vi "PH_Beckhoff.set IP and prdc Intv GUI Object.vi"(0 "VI in":refnum<vi>, 5 "error in (no error)":errorcluster) -> (14 "VI out":refnum<vi>, 19 "error out":errorcluster)   [LabVIEW 2014, in "PH_Beckhoff.lvlib"]
uses:
  PH_Beckhoff.lvlib
  CS_Core/BaseProcess/BaseProcess.lvlib
  PH_Basics/PH_Common/PH_Common.lvlib
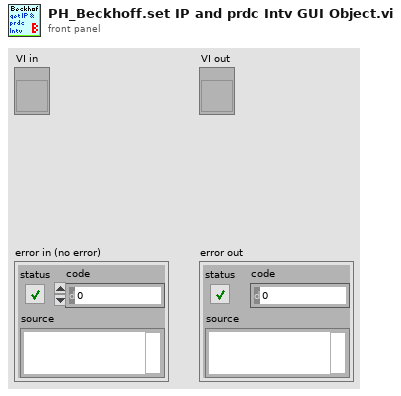
[diagram p1: front panel]
types:
  T1 = typedef "PH_Beckhoff.lvlib/PH_Beckhoff.i attribute.ctl" = cluster{"GUI Refs":T2, "operation?":bool, "Default Prdc Interval":i32, "Connection":T3, "AMS Net ID":T4, "Klemmencluster: # of":T5, "Values":T6, "IP":string, "Description":string, "configured?":bool, "Change Manager":cluster{"Detemination wanted?":bool, "Values changed at":cluster{"Sonderklemmen Inputs":i32[], "Analog Inputs":i32[], "Analog Outputs":i32[], "Digital Inputs":i32[], "Digital Outputs":i32[]}}, "Difference to handle an analog input as change":u32}
  T2 = typedef "PH_Beckhoff.lvlib/PH_Beckhoff.GUI Refs.ctl" = cluster{"ADS Error":refnum<vi>, "Values":refnum<vi>, "configured?":refnum<vi>, "Connection":refnum<vi>, "IP":refnum<vi>, "Prdc Int [ms]":refnum<vi>}
  T3 = typedef "PH_Beckhoff.lvlib/PH_Beckhoff.Connectivity.ctl" = cluster{"DLL?":bool, "Port?":bool, "Client?":bool, "Ping?":bool, "unsuccessful Pings":u32}
  T4 = typedef "Beckhoff - Driver np.lvlib/Beckhoff Access.ctl" = cluster{"DLL path":path, "AMS Net ID":cluster{"1st # of IP":u8, "2nd # of IP":u8, "3rd # of IP":u8, "4th # of IP":u8, "In Port":u8, "Out Port":u8}}
  T5 = typedef "Beckhoff - Driver np.lvlib/Klemmendeclarer.ctl" = cluster{"Offset due to Sonderklemms":u32, "analog Inputs":u32, "analog Outputs":u32, "digital Input Bits":u32, "digital Output Bits":u32}
  T6 = typedef "PH_Beckhoff.lvlib/PH_Beckhoff.Values.ctl" = cluster{"Sonderklemmen Inputs":T7, "Analog Inputs":T8, "Analog Outputs":T10, "Digital Inputs":T11, "Digital Outputs":T12}
  T7 = typedef "PH_Beckhoff.lvlib/PH_Beckhoff.Sonderklemmen Inputs.ctl" = cluster{"Total Length":u32, "Name":string, "Value":u64, "Quality":bool, "Service ID":i32, "Offset":u32, "Length":u32}[]
  T8 = typedef "PH_Beckhoff.lvlib/PH_Beckhoff.Analog Inputs.ctl" = cluster{"Name":string, "Value":u32, "Quality":bool, "Service ID":i32, "Sca Type":T9}[]
  T9 = typedef "PH_Beckhoff.lvlib/PH_Beckhoff.Scaling Type.ctl" = enum16{"none", "0 ... 15 Bit -> 0 ... 5", "0 ... 15 Bit -> 0 ... 10", "0 ... 15 Bit -> 0 ... 25", "0 ... 15 Bit -> 4 ... 20", "0 ... 15 Bit -> 0 ... 1", "0 ... 15 Bit -> 0 ... 20000", "0 ... 15 Bit -> 0 ... 24000"}
  T10 = typedef "PH_Beckhoff.lvlib/PH_Beckhoff.Analog Outputs.ctl" = cluster{"Name":string, "Value":u32, "Quality":bool, "Wanted Value":u32, "Service ID":i32, "Sca Type":T9}[]
  T11 = typedef "PH_Beckhoff.lvlib/PH_Beckhoff.Digital Inputs.ctl" = cluster{"Name":string, "Value":bool, "Quality":bool, "Service ID":i32, "inverted?":bool}[]
  T12 = typedef "PH_Beckhoff.lvlib/PH_Beckhoff.Digital Outputs.ctl" = cluster{"Name":string, "Value":bool, "Quality":bool, "Wanted Value":bool, "Service ID":i32, "inverted?":bool}[]
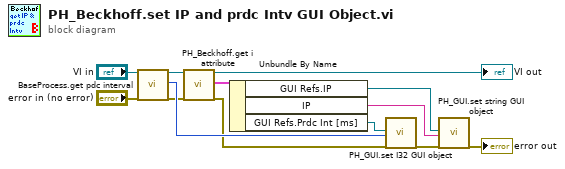
[diagram p0: block diagram]
diagram:
  n1 = call "BaseProcess.get pdc interval.vi"("i ref in"="VI in", "error in (no error)"="error in (no error)") -> ("i ref out"=w8:refnum<vi>, "PeriodicInterval"=w11:i32, "error out"=w6:errorcluster)  [unwired: 15 in]
  n2 = call "PH_Beckhoff.get i attribute.vi"("i ref in"=w8, "error in (no error)"=w6) -> ("i ref out"=→"VI out":refnum<vi>, "i attribute"=w13:T1, "error out"=w5:errorcluster)  [unwired: 15 in]
  n3 = Unbundle By Name(w13) -> ("GUI Refs.IP"=w2:refnum<vi>, "IP"=w3:string, "GUI Refs.Prdc Int [ms]"=w10:refnum<vi>)
  n4 = call "PH_GUI.set I32 GUI object.vi"("I32 GUI Ref"=w10, "value"=w11, "error in (no error)"=w5) -> ("error out"=w12:errorcluster)  [unwired: 16 in]
  n5 = call "PH_GUI.set string GUI object.vi"("GUI object Ref"=w2, "Text"=w3, "error in"=w12) -> ("error out"=→"error out":errorcluster)  [unwired: 16 in]
